vi "Info1DClusterArray22DArray.vi"(2 "error in (no error)":errorcluster caption="错误输入（无错误）", 3 "1D ClusterArray":T1[](array[typedef])=[{"得分"=1, "英雄"="as"}, {"得分"=1, "英雄"="asc"}, {"得分"=2, "英雄"="sdc"}, {"得分"=3, "英雄"="sdv"}]) -> (0 "error out":errorcluster caption="错误输出", 1 "2D StringArray":string[][](array[string]))   [LabVIEW 2019]
uses:
  ctl/InfoOfPlayer.ctl
panel:
  out "数组":string[](array[string])
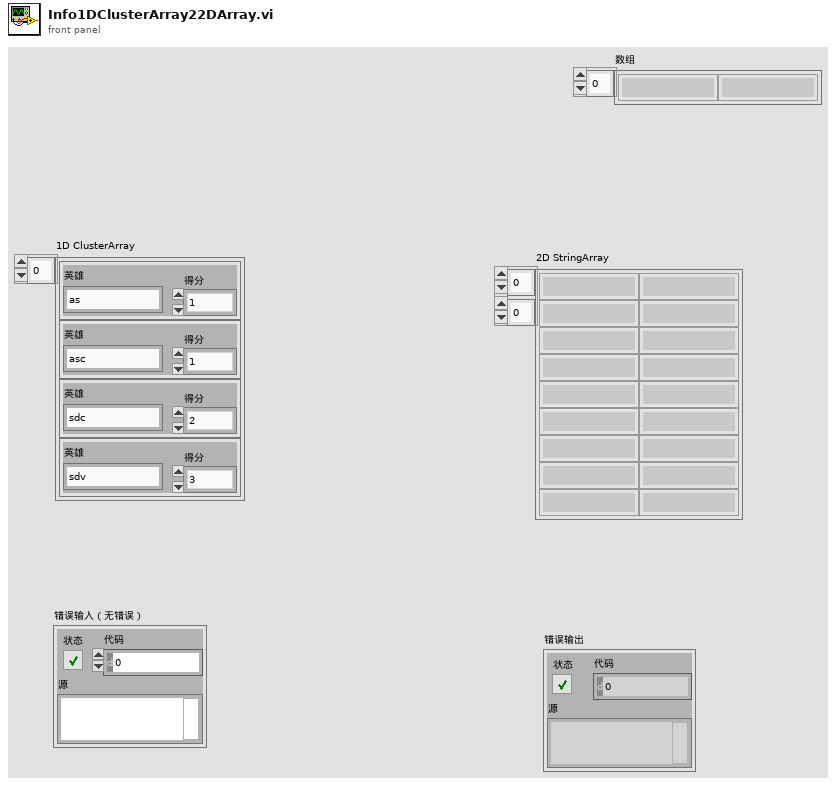
[diagram p1: front panel]
types:
  T1 = typedef "InfoOfPlayer.ctl" = cluster{"得分":i32, "英雄":string}
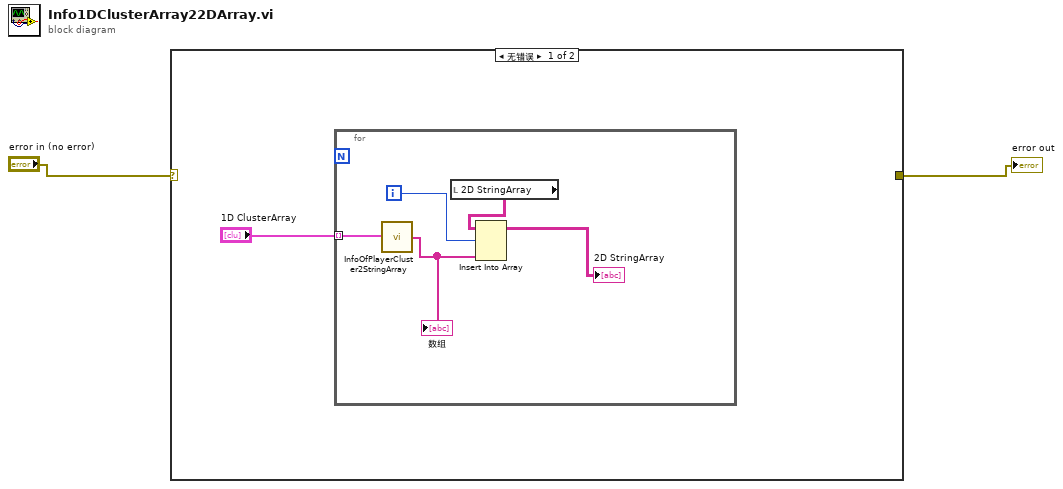
[diagram p0: block diagram]
diagram:
  n1 = case shown="无错误" "error in (no error)" {
    selector: "error in (no error)" -> [_ w9]
    tunnel: [_ w9] -> w1
    frame No Error {
      n2 = for {
        tunnel: "1D ClusterArray" -> [w8] mode=indexing
        i -> [w5]
        n3 = call "InfoOfPlayerCluster2StringArray.vi"("玩家信息"=w8) -> ("数组"=w7:string[])
        "数组" <- w7
        n4 = local read "2D StringArray"() -> (w6:string[][])
        n5 = Insert Into Array(array=w6, index (row)=w5, new element=w7) -> (→"2D StringArray":string[][])  [unwired: 1 in]
      }
    }
    frame Error {
    }
  }
  "error out" <- w1
